vi "CAN capture from cont mont cond 1.vi"() -> ()   [LabVIEW 2019]
panel:
  out "Waveform Graph":u8[](graph)
  in  "y 2":u8 format="%.0x"
  out "appended array 3":u8[][](array[numeric]) format="%.0x"
  in  "y":u32 format="%.0x"
  in  "appended array 2":u8[][](array[numeric])=array9201x8[73608 elements] format="%.0x"
  in  "appended array":u32[](array[numeric])=array[9201 elements] format="%.0x"
  # "21, 10, 2"
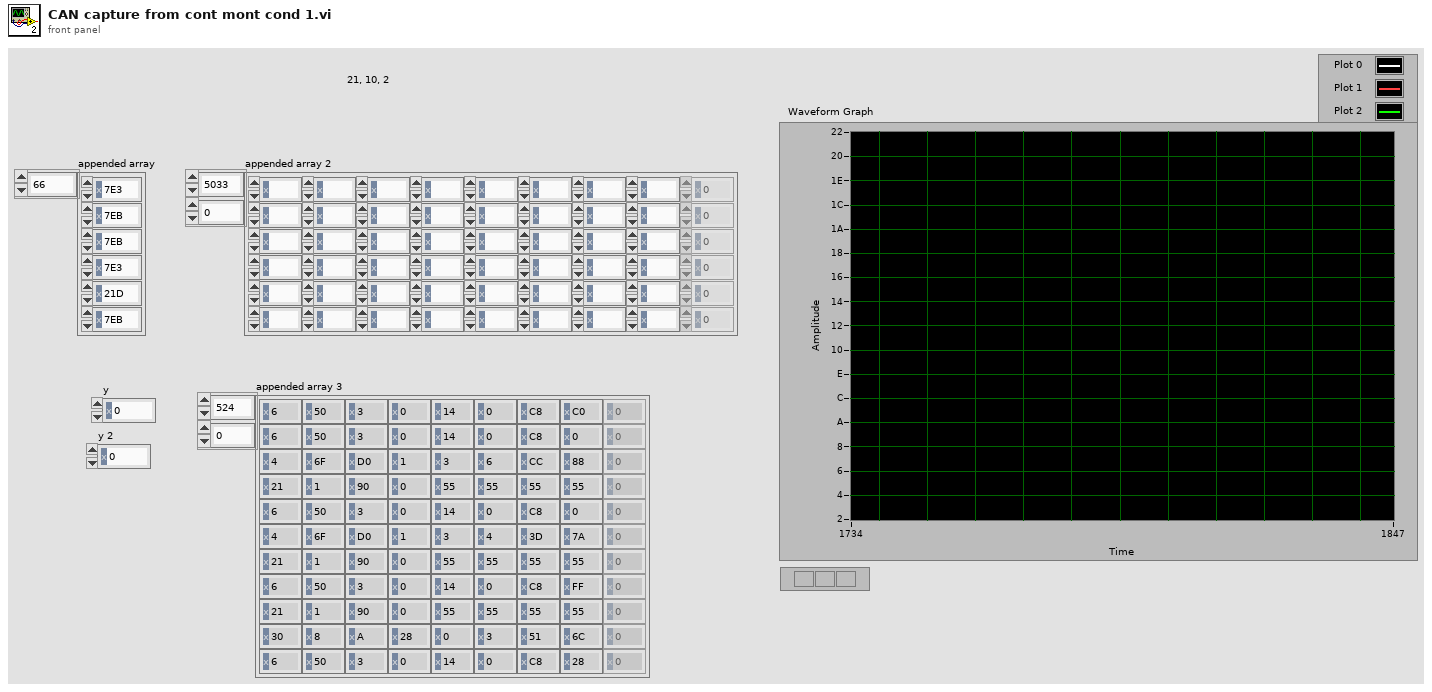
[diagram p1: front panel]
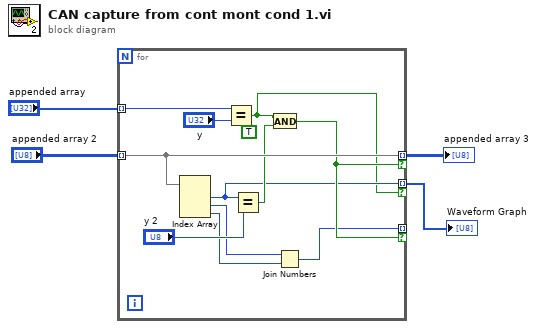
[diagram p0: block diagram]
diagram:
  n1 = for {
    tunnel: "appended array" -> [w15] mode=indexing
    tunnel: "appended array 2" -> [w13] mode=indexing
    tunnel: [w13] -> w3 mode=indexing if=w11
    tunnel: [w7] -> _ mode=indexing if=w11
    tunnel: [w6] -> w1 mode=indexing if=w5
    (unwired) TRUE ("y")
    n2 = Index Array(array=w13) -> (element #1=w6:u8, element #2=w9:u8, element #3=w8:u8)  [unwired: 3 in]
    n3 = Equal?(x=w15, y="y") -> (x = y?=w5:bool)
    n4 = Equal?(x=w6, y="y 2") -> (x = y?=w10:bool)
    n5 = And(x=w5, y=w10) -> (x .and. y?=w11:bool)
    n6 = Join Numbers(hi=w9, lo=w8) -> ((hi.lo)=w7:u16)
  }
  "appended array 3" <- w3
  "Waveform Graph" <- w1
